vi "VCS Request CAN Frame.vi"(8 "error in (no error)":errorcluster, 9 "CAN info":cluster{"cobId":u16, "length":u16}, 11 "keyHandle in":u32) -> (0 "error out":errorcluster, 2 "data":u8[](array[numeric]), 3 "keyHandle out":u32)   [LabVIEW 2010]
doc: "<B>VCS Request CAN Frame</B> requests a general CAN Frame from the CAN bus using Remote Transmit Request (RTR)."
uses:
  Resources/EposCmd.dll
  Resources/EposCmd64.dll
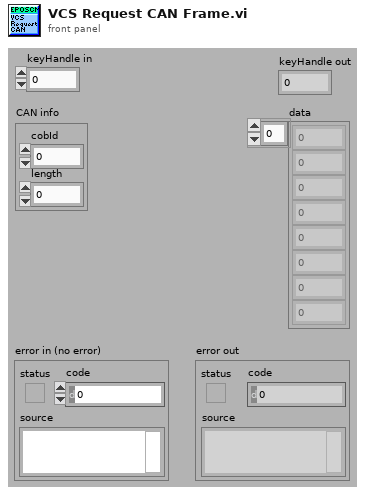
[diagram p1: front panel]
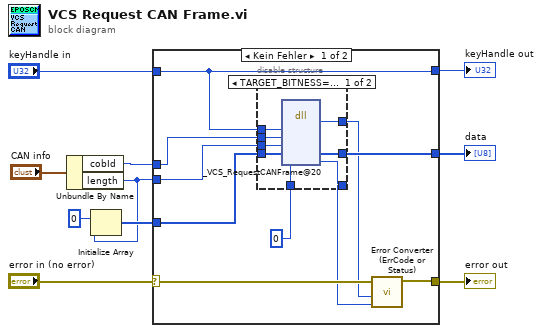
[diagram p0: block diagram]
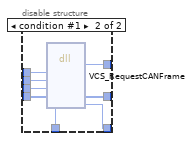
[diagram p2: hidden frame]
diagram:
  n1 = Unbundle By Name("CAN info") -> ("cobId"=w2:u16, "length"=w1:u16)
  n2 = Initialize Array(u8 0, w1) -> (w7:u8[])
  n3 = case shown="Kein Fehler" "error in (no error)" {
    selector: "error in (no error)" -> [w19 w39]
    tunnel: [w18 w39] -> w9
    tunnel: "keyHandle in" -> [w14 w37]
    tunnel: [w20 w38] -> w6
    tunnel: w7 -> [w16 w38]
    tunnel: [w14 w37] -> w4
    tunnel: w2 -> [w11 _]
    tunnel: w1 -> [w12 _]
    frame No Error {
      n4 = disable-structure shown="TARGET_BITNESS==32, Standard" {
        disable-tunnel: [w28 w36] -> w20
        disable-tunnel: [w27 w35] -> w17
        disable-tunnel: w16 -> [w26 w34]
        disable-tunnel: u32 0 ("pErrorCode") -> [w25 w33]
        disable-tunnel: w14 -> [w24 w32]
        disable-tunnel: [w23 w31] -> w13
        disable-tunnel: w12 -> [w22 w30]
        disable-tunnel: w11 -> [w21 w29]
        frame condition #0 (active) {
          n5 = dll-call lib="C:/Sources/LabView/maxon EPOS/Resources/EposCmd.*" fn="_VCS_RequestCANFrame@20"("KeyHandle"=w24, "CobID"=w21, "Length"=w22, "pData"=w26, "pErrorCode"=w25) -> (w23:i32, "pData"=w28:u8[], "pErrorCode"=w27:u32)  [unwired: 6 in, 2 out]
        }
        frame condition #1 {
          n6 = dll-call lib="C:/setup/Resources/EposCmd64.*" fn="VCS_RequestCANFrame" ("EposCmd.dll:_VCS_RequestCANFrame@20")("KeyHandle"=w32, "CobID"=w29, "Length"=w30, "pData"=w34, "pErrorCode"=w33) -> ("Rückgabetyp"=w31:i32, "pData"=w36:u8[], "pErrorCode"=w35:u32)  [unwired: 6 in, 2 out]
        }
      }
      n7 = call "Error Converter (ErrCode or Status).vi"("error code"=w17, "return type"=w13, "error in (no error)"=w19) -> ("error out"=w18:errorcluster)  [unwired: 7 in]
    }
    frame Error {
    }
  }
  "error out" <- w9
  "data" <- w6
  "keyHandle out" <- w4
